vi "getParameters.vi"(11 "ApplyAOSCorrectionByBendingModesCommand in":refnum<class "ApplyAOSCorrectionByBendingModesCommand.lvclass">) -> (2 "Parameters":T1, 3 "ApplyAOSCorrectionByBendingModesCommand out":refnum<class "ApplyAOSCorrectionByBendingModesCommand.lvclass">)   [LabVIEW 2016, in "ApplyAOSCorrectionByBendingModesCommand.lvclass"]
uses:
  ApplyAOSCorrectionByBendingModesCommand.lvclass
  DataTypes/Topics/CommandApplyAOSCorrectionByBendingModes.ctl
  DataTypes/Topics/Parts/CommandId.ctl
  ApplyAOSCorrectionByBendingModesCommand.lvclass/ApplyAOSCorrectionByBendingModesCommand.ctl
  DataTypes/Topics/M1M3SupportTopics.lvlib
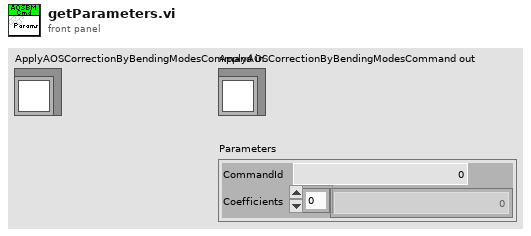
[diagram p1: front panel]
types:
  T1 = typedef "M1M3SupportTopics.lvlib/CommandApplyAOSCorrectionByBendingModes.ctl" = cluster{"CommandId":T2, "Coefficients":dbl[]}
  T2 = typedef "M1M3SupportTopics.lvlib/CommandId.ctl" = i32
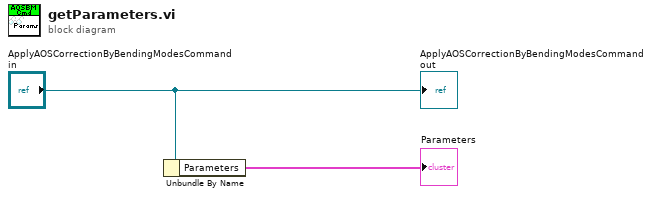
[diagram p0: block diagram]
diagram:
  n1 = Unbundle By Name("ApplyAOSCorrectionByBendingModesCommand in") -> ("Parameters"=→"Parameters":T1)
  "ApplyAOSCorrectionByBendingModesCommand out" <- "ApplyAOSCorrectionByBendingModesCommand in"
